vi "AWG Scale Standard Waveform amplitude for programming.vi"(8 "error in (no error)":errorcluster, 9 "AmpGain":i32, 10 "Waveform In":T1={"Name"="", "Waveform"={"waveform type"=enum."sine", "amplitude"=1.0, "Time"=256.0}} caption="Cluster" {"Waveform"."amplitude" min=0.0 max=1.0 format="%.2f"}, 11 "Instrument Handle In":refnum<k15>) -> (0 "error out":errorcluster, 2 "Waveform Out":T1 {"Waveform"."amplitude" min=0.0 max=1.0 format="%.2f"}, 3 "Instrument Handle Out":refnum<k15>)   [LabVIEW 2013]
doc: "This VI reads the Gain and Offset of the AWG instrument and then rescales the amplitude of the waveform accordingly to range between -1 to 1 for programming the AWG instrument."
uses:
  StandardWaveformWithName.ctl
  StandardWaveform.ctl
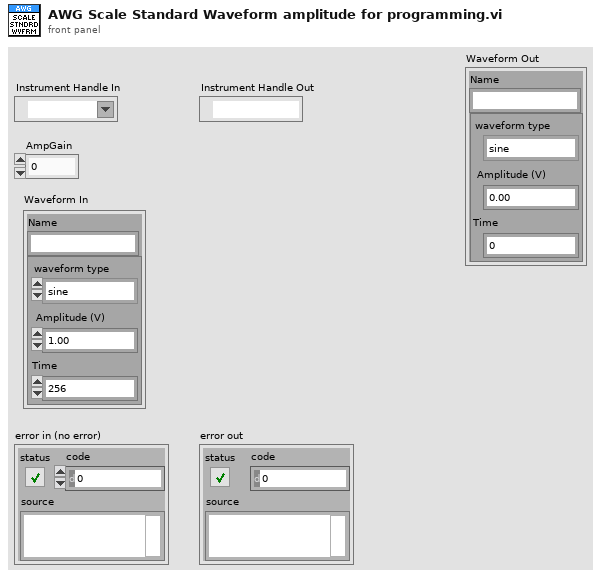
[diagram p1: front panel]
types:
  T1 = typedef "StandardWaveformWithName.ctl" = cluster{"Name":string, "Waveform":T2}
  T2 = typedef "StandardWaveform.ctl" = cluster{"waveform type":enum16{"sine", "cosine", "triangle", "square", "sawtooth", "increasing ramp", "decreasing ramp", "DC Value"}, "amplitude":dbl, "Time":dbl}
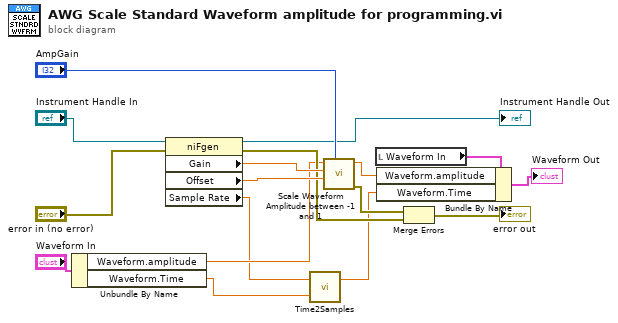
[diagram p0: block diagram]
diagram:
  n1 = Unbundle By Name("Waveform In") -> ("Waveform.amplitude"=w8:dbl, "Waveform.Time"=w2:dbl)
  n2 = property class="niFgen"(reference="Instrument Handle In", error in="error in (no error)") -> (reference out=→"Instrument Handle Out":refnum<k15>, error out=w9:errorcluster, "Gain"=w16:dbl, "Offset"=w15:dbl, "Sample Rate"=w3:dbl)
  n3 = call "Time2Samples.vi"("Time"=w2, "SampleRate"=w3) -> ("Samples"=w1:dbl)  [unwired: 1 in]
  n4 = call "Scale Waveform Amplitude between -1 and 1.vi"("AmpGain"="AmpGain", "Offset"=w15, "Gain"=w16, "Waveform Amplitude In (V)"=w8) -> ("error out"=w10:errorcluster, "Waveform Amplitude Out (-1 to 1)"=w6:dbl)  [unwired: 6 in]
  n5 = local read "Waveform In"() -> (w7:T1)
  n6 = Bundle By Name(cluster=w7, "Waveform.amplitude"=w6, "Waveform.Time"=w1) -> (→"Waveform Out":T1)
  n7 = Merge Errors(w10, w9) -> (→"error out":errorcluster)
